vi "Set JSON Data.vi"(7 "VI Reference":refnum<vi>, 8 "error in (no error)":errorcluster, 10 "Value":string, 11 "String In":refnum<class "String.lvclass">) -> (0 "error out":errorcluster, 3 "String Out":refnum<class "String.lvclass">)   [LabVIEW 2017, in "Front Panel Publisher.lvlib" / "String.lvclass"]
uses:
  String.lvclass
  Object_class/Object.lvclass
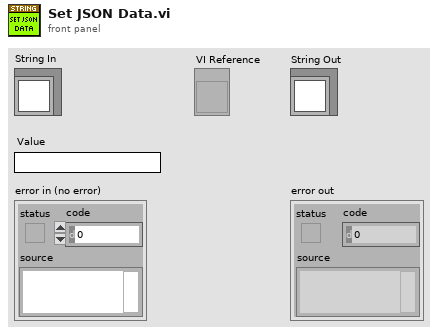
[diagram p1: front panel]
types:
  T1 = typedef "Front Panel Publisher.lvlib/Object.lvclass/Attributes.ctl" = cluster{"UID":i32, "Type":string, "Starting Location":T2, "Reference":refnum<vi>, "Cluster Component":bool, "Starting Rect Position":cluster{"Left":i16, "Top":i16}, "Owning Pane":refnum<vi>, "Master Total Rect Delta":T3}
  T2 = typedef "Front Panel Publisher.lvlib/Object.lvclass/Coordinates.ctl" = cluster{"Left":i32, "Top":i32, "Height":u32, "Width":u32}
  T3 = typedef "LVRectTypeDef.ctl" = cluster{"Left":i16, "Top":i16, "Right":i16, "Bottom":i16}
  T4 = typedef "Front Panel Publisher.lvlib/String.lvclass/Attributes.ctl" = cluster{"String Is Path":bool}
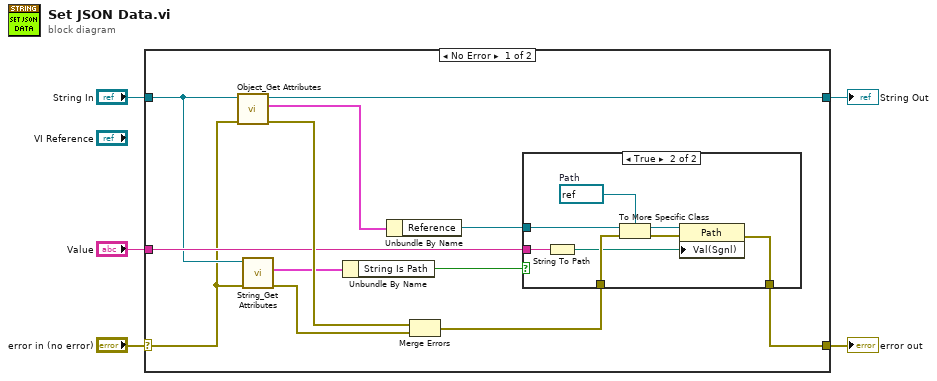
[diagram p0: block diagram]
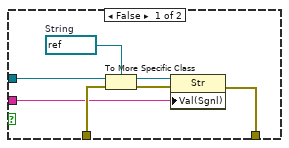
[diagram p2: hidden frame]
diagram:
  n1 = case shown="No Error" "error in (no error)" {
    selector: "error in (no error)" -> [w6 w34]
    tunnel: [w17 w34] -> w4
    tunnel: [w14 w33] -> w2
    tunnel: "String In" -> [w11 w33]
    tunnel: "Value" -> [w12 _]
    frame No Error {
      n2 = call "Object_Get Attributes.vi"("error in (no error)"=w6, "Object In"=w11) -> ("error out"=w16:errorcluster, "Object Attributes"=w15:T1, "Object Out"=w14:refnum<class "String.lvclass">)  [unwired: 7 in]
      n3 = call "String_Get Attributes.vi"("error in (no error)"=w6, "String In"=w11) -> ("error out"=w7:errorcluster, "String Attributes"=w10:T4)  [unwired: 7 in, 1 out]
      n4 = Unbundle By Name(w10) -> ("String Is Path"=w9:bool)
      n5 = Unbundle By Name(w15) -> ("Reference"=w13:refnum<vi>)
      n6 = Merge Errors(w16, w7) -> (w8:errorcluster)
      n7 = case shown="True" w9 {
        tunnel: [w24 w32] -> w17
        tunnel: w8 -> [w23 w31]
        tunnel: w13 -> [w21 w29]
        tunnel: w12 -> [w20 w28]
        frame False {
          w18 = refnum<vi> refnum  # String
          n8 = To More Specific Class(target class=w18, reference=w21, error in=w23) -> (specific class reference=w19:refnum<vi>, error out=w22:errorcluster)
          n9 = property class="Str"(reference=w19, error in=w22, "Val(Sgnl)"=w20) -> (error out=w24:errorcluster)  [unwired: 1 out]
        }
        frame True {
          w26 = refnum<vi> refnum  # Path
          n10 = String To Path(string=w28) -> (path=w25:path)
          n11 = To More Specific Class(target class=w26, reference=w29, error in=w31) -> (specific class reference=w27:refnum<vi>, error out=w30:errorcluster)
          n12 = property class="Path"(reference=w27, error in=w30, "Val(Sgnl)"=w25) -> (error out=w32:errorcluster)  [unwired: 1 out]
        }
      }
    }
    frame Error {
    }
  }
  "error out" <- w4
  "String Out" <- w2
